vi "Load Settings from XML.vi"(8 "error in (no error)":errorcluster, 11 "Settings in":T1={"Logging Configuration"={"Log File Base Path"=path "", "Max Samples"=0, "File Refnum"=refnum, "Log Piezo"=FALSE, "Piezo File Refnum"=refnum, "Log Capacitive"=FALSE, "Cap File Refnum"=refnum, "Filename"="", "Path where to save"=path ""}, "Piezo Config"={"Piezo Serial Number"=41848555, "MG17Piezo"=refnum, "Setpoint (um)"=0.0}, "Capacitive Config"={"IP Address"="192.168.168.57", "Handle"=0, "Refresh Time (ms)"=0.0}, "Hardware Config"={"Data Source"=0, "Counter Configuration"={"DAQmx Task"="", "Counter(s)"="Dev2/ctr0", "samples per readout"=100}, "ADC Configuration"={"DAQmx Task"="", "Channel(s)"="Dev2/ctr0", "samples per readout"=100, "Sample Rate (s/s)"=100, "Max Voltage"=100.0, "Min Voltage"=100.0}}} {"Hardware Config"."Data Source" items=["Counter", "ADC"]}) -> (0 "error out":errorcluster, 3 "Settings out":T1={"Logging Configuration"={"Log File Base Path"=path "", "Max Samples"=0, "File Refnum"=refnum, "Log Piezo"=FALSE, "Piezo File Refnum"=refnum, "Log Capacitive"=FALSE, "Cap File Refnum"=refnum, "Filename"="", "Path where to save"=path ""}, "Piezo Config"={"Piezo Serial Number"=41848555, "MG17Piezo"=refnum, "Setpoint (um)"=0.0}, "Capacitive Config"={"IP Address"="192.168.168.57", "Handle"=0, "Refresh Time (ms)"=0.0}, "Hardware Config"={"Data Source"=0, "Counter Configuration"={"DAQmx Task"="", "Counter(s)"="Dev2/ctr0", "samples per readout"=100}, "ADC Configuration"={"DAQmx Task"="", "Channel(s)"="Dev2/ctr0", "samples per readout"=100, "Sample Rate (s/s)"=100, "Max Voltage"=100.0, "Min Voltage"=100.0}}} {"Hardware Config"."Data Source" items=["Counter", "ADC"]})   [LabVIEW 2013, in "Settings.lvlib"]
doc: "Attempts to load previous user specified settings from an XML file.\n\nThis VI will not generate an error. If a suitable XML file can't be loaded and parsed then it will simply return the default settings."
uses:
  Settings.lvlib
  Settings.ctl
  Logging/Logging Configuration.ctl
  Piezo/Hardware Configuration.ctl
  Capacitive/Hardware Configuration.ctl
  Acquisition/Hardware Configuration.ctl
  Acquisition/Counter Configuration.ctl
  ADC/ADC Configuration.ctl
  <vilib>/Utility/xml.llb/Read From XML File(string).vi
  <vilib>/Utility/xml.llb/Write to XML File(string).vi
  Acquisition/Acquisition.lvlib
  Logging/Logging.lvlib
  Piezo/Piezo.lvlib
  Capacitive/Capacitive.lvlib
panel:
  # "(Scroll up for Settings Controls)"
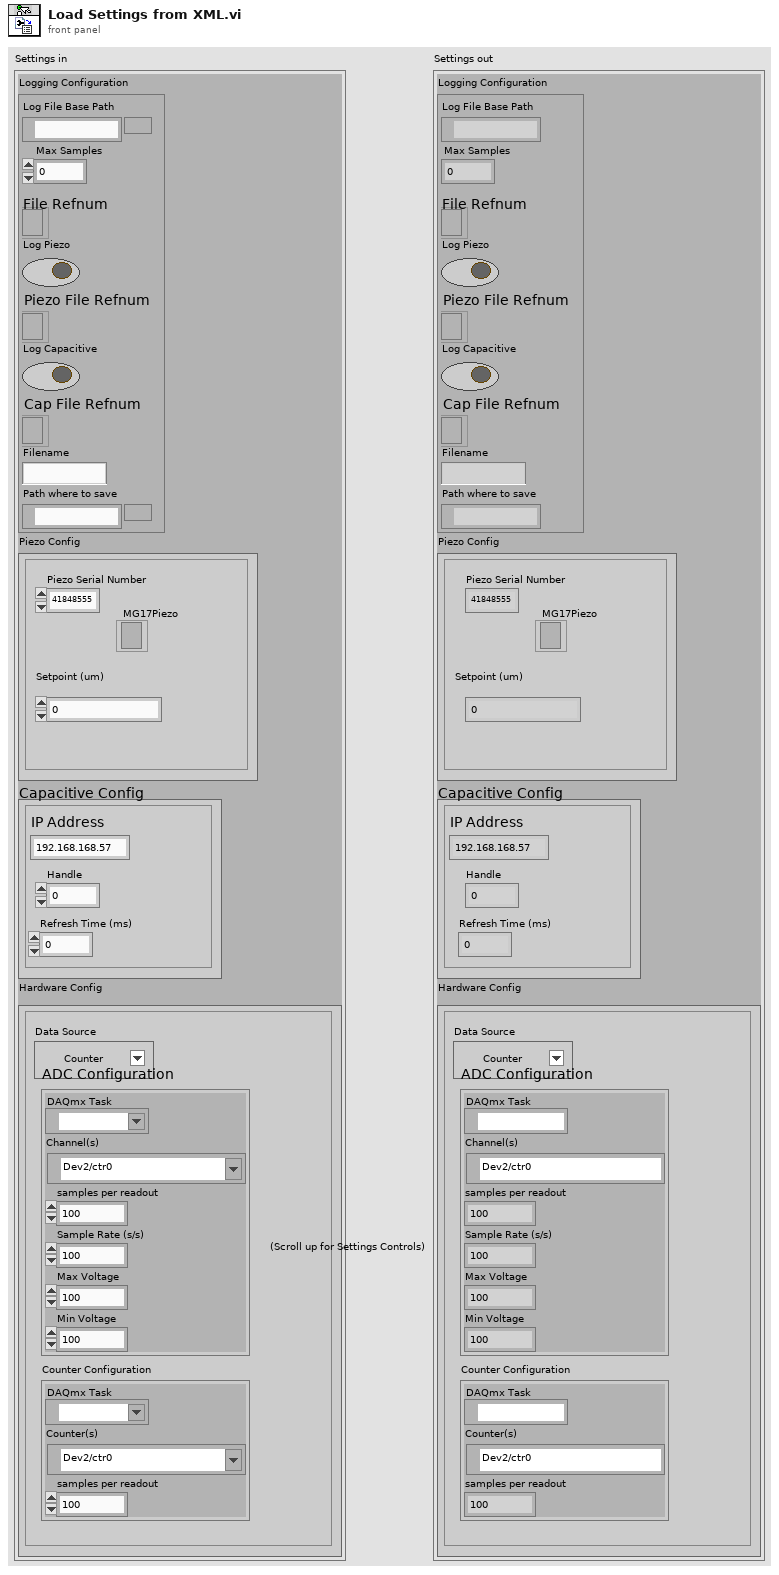
[diagram p1: front panel]
types:
  T1 = typedef "Settings.lvlib/Settings.ctl" = cluster{"Logging Configuration":T2, "Piezo Config":T3, "Capacitive Config":T4, "Hardware Config":T5}
  T2 = typedef "Logging.lvlib/Logging Configuration.ctl" = cluster{"Log File Base Path":path, "Max Samples":u32, "File Refnum":refnum<file>, "Log Piezo":bool, "Piezo File Refnum":refnum<file>, "Log Capacitive":bool, "Cap File Refnum":refnum<file>, "Filename":string, "Path where to save":path}
  T3 = typedef "Piezo.lvlib/Hardware Configuration.ctl" = cluster{"Piezo Serial Number":i32, "MG17Piezo":refnum<k7>, "Setpoint (um)":sgl}
  T4 = typedef "Capacitive.lvlib/Hardware Configuration.ctl" = cluster{"IP Address":string, "Handle":u32, "Refresh Time (ms)":dbl}
  T5 = typedef "Acquisition.lvlib/Hardware Configuration.ctl" = cluster{"Data Source":u16, "Counter Configuration":T6, "ADC Configuration":T7}
  T6 = typedef "Acquisition.lvlib/Counter Configuration.ctl" = cluster{"DAQmx Task":refnum<k21>, "Counter(s)":tag, "samples per readout":i32}
  T7 = typedef "Acquisition.lvlib/ADC Configuration.ctl" = cluster{"DAQmx Task":refnum<k21>, "Channel(s)":tag, "samples per readout":i32, "Sample Rate (s/s)":i32, "Max Voltage":dbl, "Min Voltage":dbl}
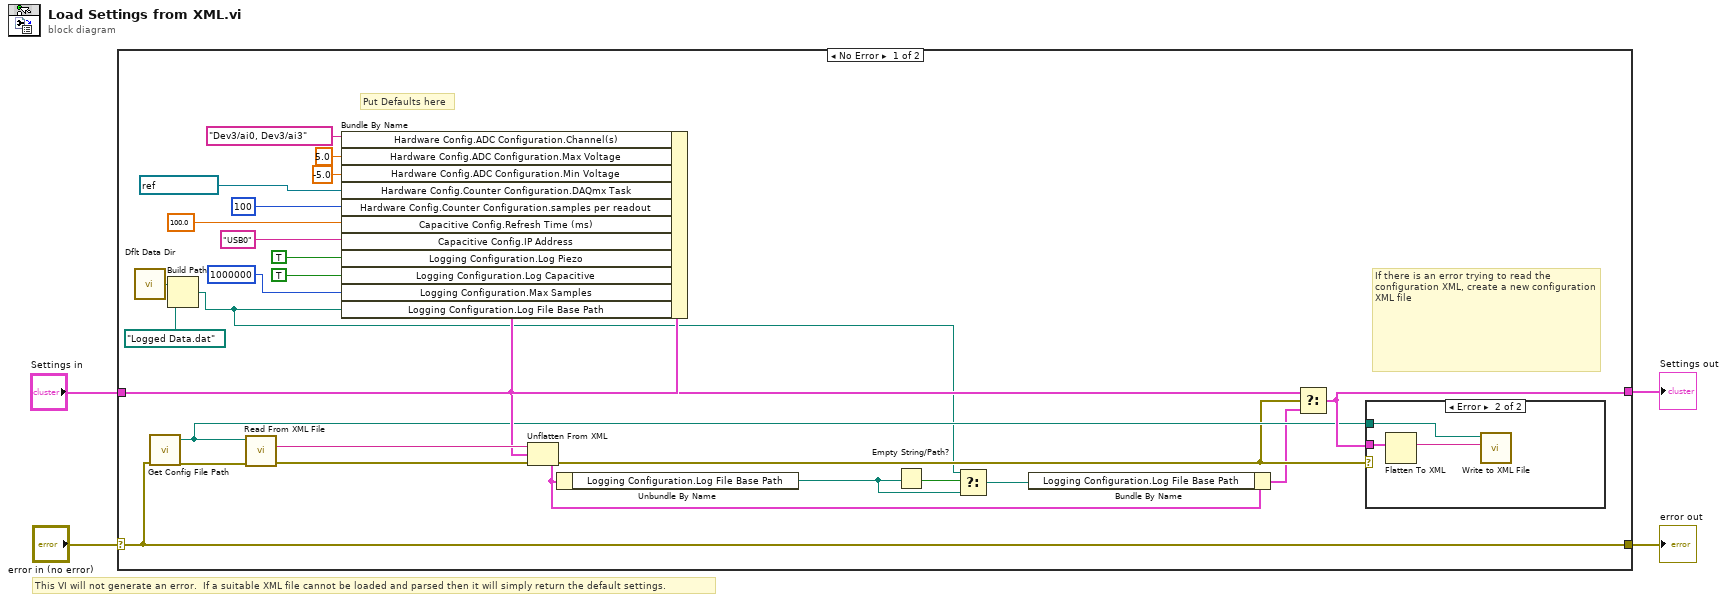
[diagram p0: block diagram]
diagram:
  # "This VI will not generate an error.  If a suitable XML file cannot be loaded and parsed then it will simply return the default settings."
  n1 = case shown="No Error" "error in (no error)" {
    selector: "error in (no error)" -> [w29 w36]
    tunnel: [w29 w36] -> w3
    tunnel: "Settings in" -> [w28 w35]
    tunnel: [w24 w35] -> w1
    frame No Error {
      # "Put Defaults here"
      # "If there is an error trying to read the configuration XML, create a new configuration XML file"
      n2 = call <vilib>:"Dflt Data Dir.vi"() -> ("App:Default Data Directory"=w26:path)
      n3 = call "Get Config File Path.vi"("error in (no error)"=w29) -> ("error out"=w31:errorcluster, "XML File Path"=w23:path)  [unwired: 9 in]
      n4 = Build Path(base path=w26, name or relative path=path "Logged Data.dat" ("App:Default Data Directory")) -> (appended path=w19:path)
      n5 = call-poly <vilib>:"Read From XML File.vi"("error in (no error)"=w31, "XML File Path"=w23) -> ("error out"=w22:errorcluster, "XML Elements"=w30:string)  [unwired: 7 in, 1 out]
      n6 = Bundle By Name(cluster=w28, "Hardware Config.ADC Configuration.Channel(s)"=tag "Dev3/ai0, Dev3/ai3", "Hardware Config.ADC Configuration.Max Voltage"=5.0, "Hardware Config.ADC Configuration.Min Voltage"=-5.0, "Hardware Config.Counter Configuration.DAQmx Task"=refnum<k21> "Dev2/ctr0" ("Hardware Configuration.DAQmx Task"), "Hardware Config.Counter Configuration.samples per readout"=100 ("Hardware Configuration.samples per readout"), "Capacitive Config.Refresh Time (ms)"=100.0, "Capacitive Config.IP Address"="USB0", "Logging Configuration.Log Piezo"=TRUE, "Logging Configuration.Log Capacitive"=TRUE, "Logging Configuration.Max Samples"=u32 1000000, "Logging Configuration.Log File Base Path"=w19) -> (w27:T1)
      n7 = Unflatten From XML(xml string=w30, type=w27, error in (no error)=w22) -> (value=w17:T1, error out=w21:errorcluster)
      n8 = Unbundle By Name(w17) -> ("Logging Configuration.Log File Base Path"=w15:path)
      n9 = Empty String/Path?(string/path=w15) -> (empty?=w20:bool)
      n10 = Select(t=w19, s=w20, f=w15) -> (s? t:f=w18:path)
      n11 = Bundle By Name(cluster=w17, "Logging Configuration.Log File Base Path"=w18) -> (w16:T1)
      n12 = Select(t=w27, s=w21, f=w16) -> (s? t:f=w24:T1)
      n13 = case shown="Error" w21 {
        tunnel: w24 -> [_ w34]
        tunnel: w23 -> [_ w32]
        frame No Error {
        }
        frame Error {
          n14 = Flatten To XML(anything=w34) -> (xml string=w33:string)
          n15 = call-poly <vilib>:"Write to XML File.vi"("XML Input"=w33, "XML File Path"=w32) -> ()  [unwired: 7 in, 3 out]
        }
      }
    }
    frame Error {
    }
  }
  "error out" <- w3
  "Settings out" <- w1
